vi "Launch_Async_Email.vi"() -> (0 "error out":errorcluster)   [LabVIEW 2010]
uses:
  Globals/Constants_global.vi
  Email_transfer_global.vi
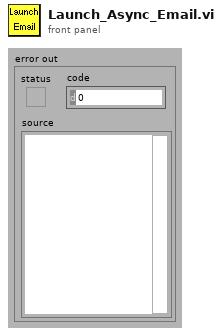
[diagram p1: front panel]
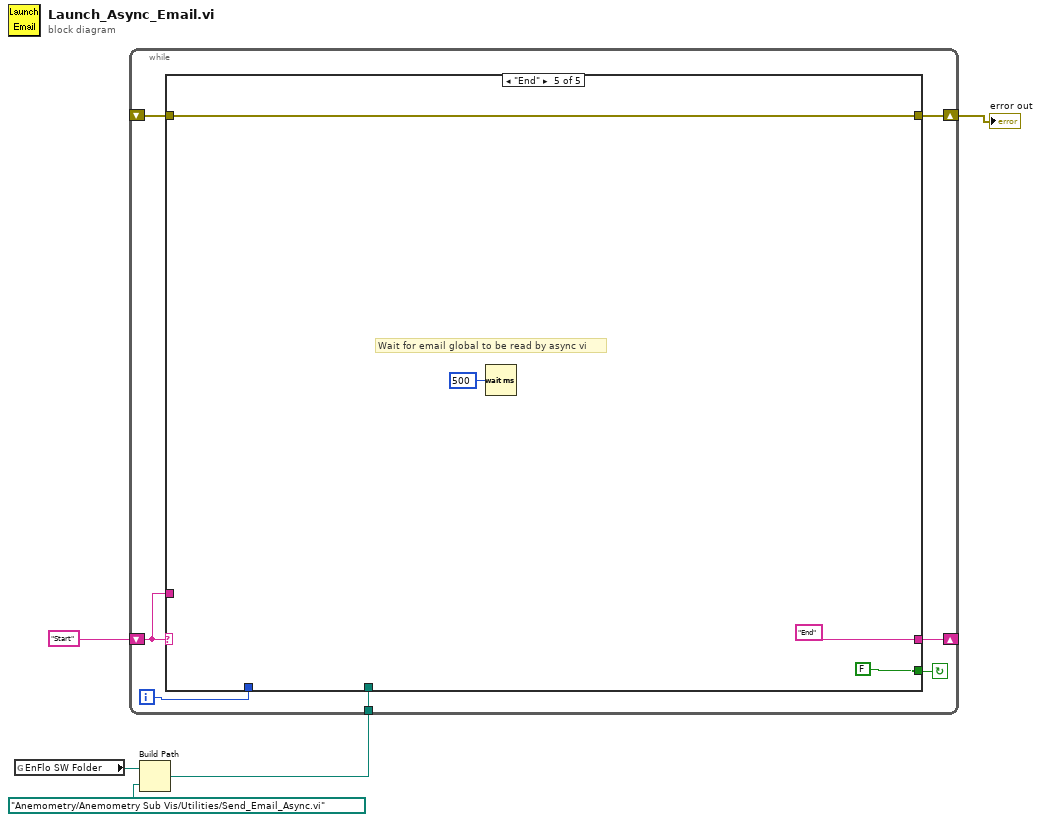
[diagram p0: block diagram]
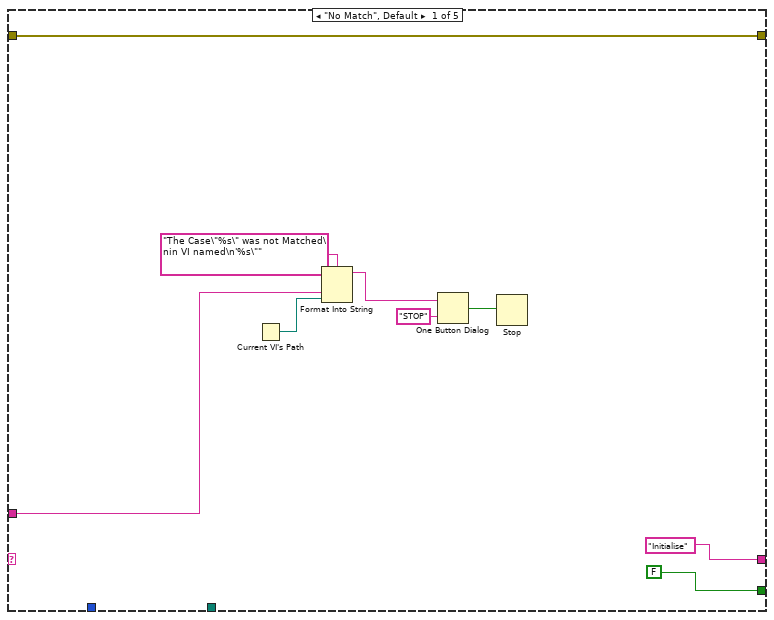
[diagram p2: hidden frame]
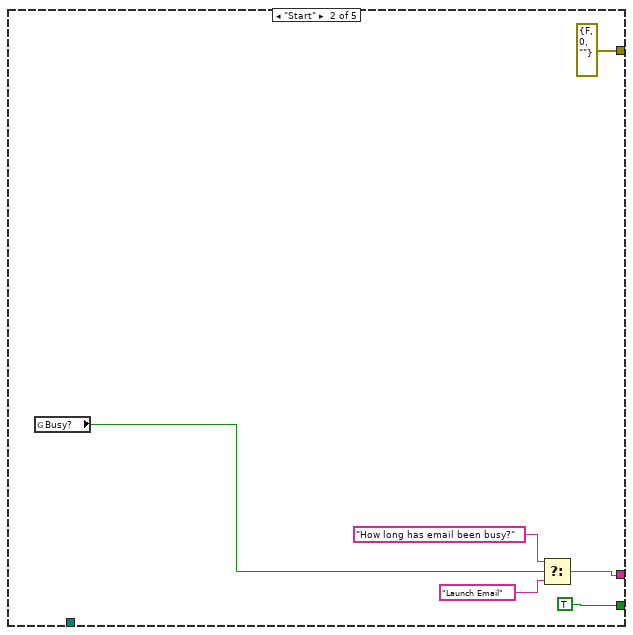
[diagram p3: hidden frame]
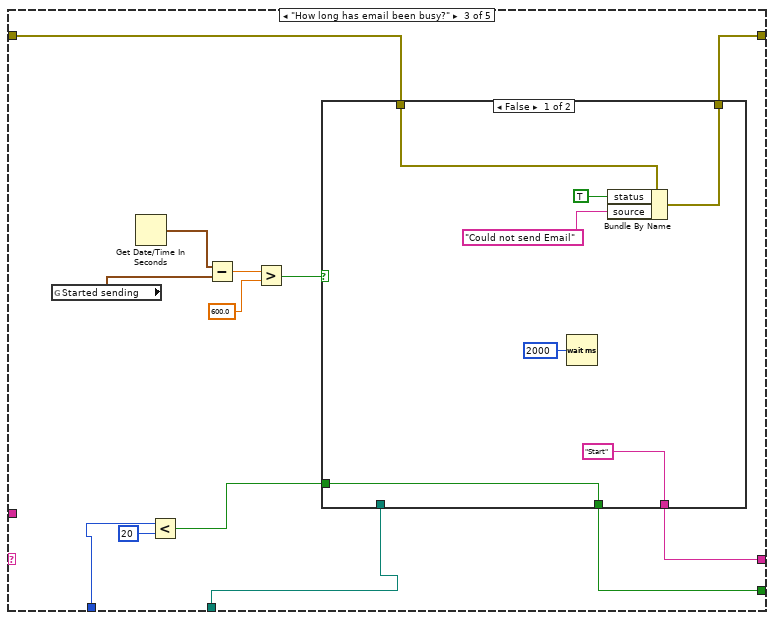
[diagram p4: hidden frame]
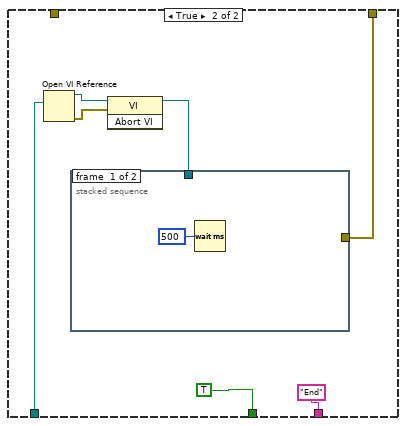
[diagram p5: hidden frame]
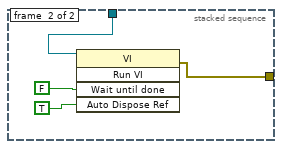
[diagram p6: hidden frame]
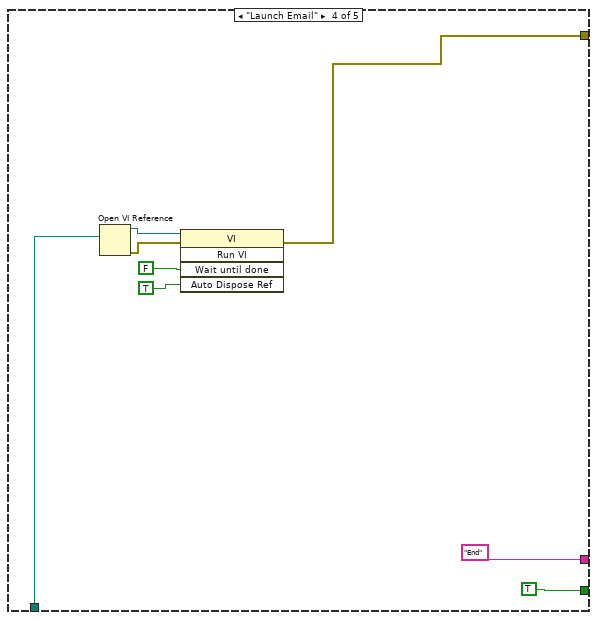
[diagram p7: hidden frame]
diagram:
  n1 = global read "Constants_global.vi" "EnFlo SW Folder"() -> (w3:path)
  n2 = Build Path(base path=w3, name or relative path=path "Anemometry/Anemometry Sub Vis/Utilities/Send_Email_Async.vi") -> (appended path=w2:path)
  n3 = while {
    shift-left: "Start" -> [w10]
    shift-right: [w11] -> _
    tunnel: w2 -> [w9]
    shift-right: [w8] -> w1
    shift-left: _ -> [w7]
    i -> [w6]
    stop <- w12 continue-if-true
    n4 = case shown="\"End\"" w10 {
      tunnel: [FALSE TRUE w33 TRUE FALSE] -> w12
      tunnel: ["Initialise" w23 w34 "End" "End"] -> w11
      tunnel: w10 -> [w16 _ _ _ _]
      tunnel: w9 -> [_ _ w35 w61 _]
      tunnel: [w13 errorcluster {"status"=FALSE, "code"=0, "source"=""} ("error out") w29 w60 w68] -> w8
      tunnel: w7 -> [w13 _ w28 _ w68]
      tunnel: w6 -> [_ _ w32 _ _]
      frame "No Match", Default {
        n5 = Current VI's Path() -> (path=w15:path)
        n6 = Format Into String(format string="The Case\"%s\" was not Matched\nin VI named\n'%s\"" ("Format String"), w16, w15) -> (resulting string=w19:string)  [unwired: 2 in, 1 out]
        n7 = One Button Dialog(message=w19, button name ("OK")="STOP") -> (true=w17:bool)
        n8 = Stop(stop? (T)=w17) -> ()
      }
      frame "Start" {
        n9 = global read "Email_transfer_global.vi" "Busy?"() -> (w25:bool)
        n10 = Select(t="How long has email been busy?", s=w25, f="Launch Email") -> (s? t:f=w23:string)
      }
      frame "How long has email been busy?" {
        n11 = global read "Email_transfer_global.vi" "Started sending"() -> (w39:timestamp)
        n12 = Get Date/Time In Seconds() -> (seconds since 1Jan1904=w40:timestamp)
        n13 = Less?(x=w32, y=20) -> (x < y?=w30:bool)
        n14 = Subtract(x=w40, y=w39) -> (x-y=w38:dbl)
        n15 = Greater?(x=w38, y=600.0) -> (0:w36:bool)
        n16 = case shown="False" w36 {
          tunnel: w35 -> [_ w52]
          tunnel: ["Start" "End"] -> w34
          tunnel: [w45 TRUE] -> w33
          tunnel: w30 -> [w45 _]
          tunnel: [w43 w49] -> w29
          tunnel: w28 -> [w44 _]
          frame False {
            n17 = Wait (ms)(milliseconds to wait=u32 2000) -> ()  [unwired: 1 out]
            n18 = Bundle By Name(cluster=w44, "status"=TRUE, "source"="Could not send Email") -> (w43:errorcluster)
          }
          frame True {
            n19 = Open VI Reference(vi path=w52) -> (vi reference=w53:refnum<vi>, error out=w54:errorcluster)  [unwired: 1 in, 4 out]
            n20 = invoke class="VI" method="Abort VI"(reference=w53, error in=w54) -> (reference out=w48:refnum<vi>)  [unwired: 1 in, 2 out]
            n21 = stacked-sequence {
              tunnel: [_ w56] -> w49
              tunnel: w48 -> [_ w57]
              frame #0 {
                n22 = Wait (ms)(milliseconds to wait=u32 500) -> ()  [unwired: 1 out]
              }
              frame #1 {
                n23 = invoke class="VI" method="Run VI"(reference=w57, "Wait until done"=FALSE, "Auto Dispose Ref"=TRUE) -> (error out=w56:errorcluster)  [unwired: 2 in, 4 out]
              }
            }
          }
        }
      }
      frame "Launch Email" {
        n24 = Open VI Reference(vi path=w61) -> (vi reference=w64:refnum<vi>, error out=w65:errorcluster)  [unwired: 1 in, 4 out]
        n25 = invoke class="VI" method="Run VI"(reference=w64, error in=w65, "Wait until done"=FALSE, "Auto Dispose Ref"=TRUE) -> (error out=w60:errorcluster)  [unwired: 1 in, 4 out]
      }
      frame "End" {
        # "Wait for email global to be read by async vi"
        n26 = Wait (ms)(milliseconds to wait=u32 500) -> ()  [unwired: 1 out]
      }
    }
  }
  "error out" <- w1
